vi "Recirc Pump Control.vi"(0 "GEA2 Reference In":refnum<k24>, 5 "Standalone?":bool, 7 "Drain Pump State":enum16{"OFF", "ON"}(ring), 11 "Error In":errorcluster) -> (4 "GEA2 Reference Out":refnum<k24>, 15 "Error Out":errorcluster)   [LabVIEW 2016, in "TL27.lvlib"]
uses:
  Projects/TL27.lvlib
  C:/Automation/DLLs/PC Dot Net/GeaCommunication.dll
  Common/LabVIEW GEA2 Toolkit/LabVIEW_GEA2_Toolkit.lvlibp/type defs/ERD Write Data In.ctl
  Common/LabVIEW GEA2 Toolkit/LabVIEW_GEA2_Toolkit.lvlibp/type defs/Data Type.ctl
  Common/LabVIEW GEA2 Toolkit/LabVIEW_GEA2_Toolkit.lvlibp/type defs/Source_Destination.ctl
  Common/LabVIEW GEA2 Toolkit/LabVIEW_GEA2_Toolkit.lvlibp
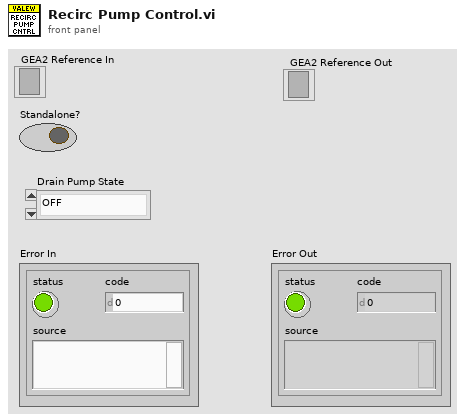
[diagram p1: front panel]
types:
  T1 = typedef "LabVIEW_GEA2_Toolkit.lvlibp/Source_Destination.ctl" = cluster{"Source":u8, "Destination":u8}
  T2 = typedef "LabVIEW_GEA2_Toolkit.lvlibp/ERD Write Data In.ctl" = cluster{"ERD Number":u16, "Data Type":T3, "Data":string}
  T3 = typedef "LabVIEW_GEA2_Toolkit.lvlibp/Data Type.ctl" = enum16{"string", "boolean", "uint8_t", "uint16_t", "uint32_t", "uint64_t", "int8_t", "int16_t", "int32_t", "int64_t"}
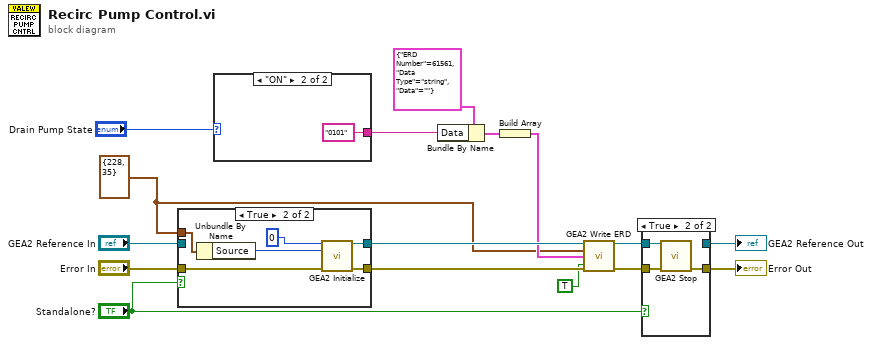
[diagram p0: block diagram]
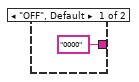
[diagram p4: hidden frame]
diagram:
  w2 = T1 {"Source"=228, "Destination"=35} ("GEA Inputs")
  n1 = case shown="True" "Standalone?" {
    tunnel: "Error In" -> [w17 w24]
    tunnel: [w17 w23] -> w16
    tunnel: "GEA2 Reference In" -> [w18 _]
    tunnel: [w18 w22] -> w11
    tunnel: w2 -> [_ w20]
    frame False {
    }
    frame True {
      n2 = Unbundle By Name(w20) -> ("Source"=w21:u8)
      n3 = call "GEA2 Initialize.vi"("Board Index"=0, "Source Address"=w21, "error in"=w24) -> ("GEA2 Reference Out"=w22:refnum<k24>, "error out"=w23:errorcluster)  [unwired: 10 in, 1 out]
    }
  }
  n4 = case shown="\"ON\"" "Drain Pump State" {
    tunnel: ["0000" "0101"] -> w7
    frame "OFF", Default {
    }
    frame "ON" {
    }
  }
  n5 = Bundle By Name(cluster=T2 {"ERD Number"=61561, "Data Type"=enum."string", "Data"=""} ("ERD Write Data In"), "Data"=w7) -> (w9:T2)
  n6 = Build Array(w9) -> (w8:T2[])
  n7 = call "GEA2 Write ERD.vi"("GEA2 Reference In"=w11, "GEA Inputs"=w2, "Write ERD List"=w8, "Error In"=w16, "Verify ERD Response?"=TRUE) -> ("GEA2 Reference Out"=w4:refnum<k24>, "Error Out"=w3:errorcluster)  [unwired: 8 in, 1 out]
  n8 = case shown="True" "Standalone?" {
    tunnel: w3 -> [w27 w31]
    tunnel: [w27 w30] -> w14
    tunnel: w4 -> [w28 w29]
    tunnel: [w28 _] -> w12
    frame False {
    }
    frame True {
      n9 = call "GEA2 Stop.vi"("GEA2 Reference In"=w29, "Error In"=w31) -> ("Error Out"=w30:errorcluster)  [unwired: 13 in]
    }
  }
  "Error Out" <- w14
  "GEA2 Reference Out" <- w12
